vi "MT_Abs.vi"(0 "X轴位置(mm)":dbl, 1 "Y轴位置(mm)":dbl, 3 "Error In":errorcluster caption="错误输入") -> (10 "Error Out":errorcluster caption="错误输出")   [LabVIEW 2020]
uses:
  lib/MT/MT_API.lvlib
panel:
  # "将设备移动到指定位置\n并等待其移动完成"
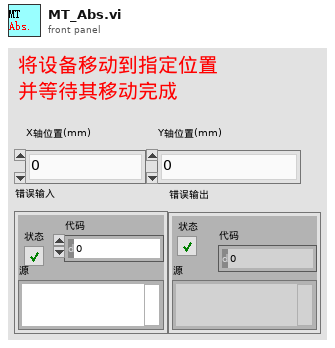
[diagram p1: front panel]
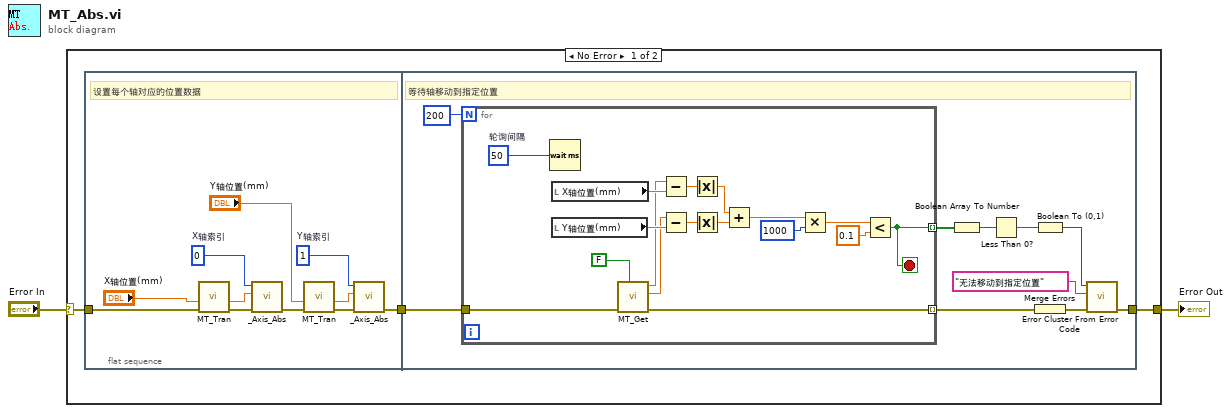
[diagram p0: block diagram]
diagram:
  n1 = case shown="No Error" "Error In" {
    selector: "Error In" -> [w5 w44]
    tunnel: [w3 w44] -> w1
    frame No Error {
      n2 = flat-sequence {
        tunnel: w5 -> [w9]
        tunnel: [w10] -> w4
        tunnel: w4 -> [w26]
        tunnel: [w21] -> w3
        frame #0 {
          w7 = 1  # Y轴索引
          w8 = 0  # X轴索引
          # "设置每个轴对应的位置数据"
          n3 = call "MT_Tran.vi"("Error In"=w9, "位置(mm)"="X轴位置(mm)") -> ("Error Out"=w12:errorcluster, "脉冲位置"=w15:dbl)  [unwired: 6 in, 2 out]
          n4 = call "_Axis_Abs.vi"("Error In"=w12, "绝对位置"=w15, "轴序号"=w8) -> ("Error Out"=w6:errorcluster)  [unwired: 8 in]
          n5 = call "MT_Tran.vi"("Error In"=w6, "位置(mm)"="Y轴位置(mm)") -> ("Error Out"=w11:errorcluster, "脉冲位置"=w13:dbl)  [unwired: 6 in, 2 out]
          n6 = call "_Axis_Abs.vi"("Error In"=w11, "绝对位置"=w13, "轴序号"=w7) -> ("Error Out"=w10:errorcluster)  [unwired: 8 in]
        }
        frame #1 {
          # "等待轴移动到指定位置"
          n7 = for {
            N: 200 -> [_]
            tunnel: w26 -> [w43]
            tunnel: [w35] -> w25 mode=indexing
            tunnel: [w34] -> w23 mode=indexing
            stop <- w35 stop-if-true
            w33 = 50  # 轮询间隔
            n8 = Wait (ms)(milliseconds to wait=w33) -> ()  [unwired: 1 out]
            n9 = local read "X轴位置(mm)"() -> (w42:dbl)
            n10 = local read "Y轴位置(mm)"() -> (w37:dbl)
            n11 = call "MT_Get.vi"("手动操作(False)"=FALSE, "Error In"=w43) -> ("Error Out"=w34:errorcluster, "Y轴位置"=w27:dbl, "X轴位置"=w28:dbl)  [unwired: 5 in, 2 out]
            n12 = Subtract(x=w28, y=w42) -> (x-y=w40:dbl)
            n13 = Subtract(x=w27, y=w37) -> (x-y=w39:dbl)
            n14 = Absolute Value(x=w40) -> (abs(x)=w41:dbl)
            n15 = Absolute Value(x=w39) -> (abs(x)=w38:dbl)
            n16 = Add(x=w41, y=w38) -> (x+y=w31:dbl)
            n17 = Multiply(x=w31, y=1000) -> (x*y=w29:dbl)
            n18 = Less?(x=w29, y=0.1) -> (x < y?=w35:bool)
          }
          n19 = Boolean Array To Number(Boolean array=w25) -> (number=w20:u32)
          n20 = Less Than 0?(x=w20) -> (x < 0?=w19:bool)
          n21 = Boolean To (0,1)(Boolean=w19) -> (0, 1=w18:i16)
          n22 = Merge Errors(w23) -> (w22:errorcluster)
          n23 = call <vilib>:"Error Cluster From Error Code.vi"("error in (no error)"=w22, "error message (\"\")"="无法移动到指定位置", "error code (0)"=w18) -> ("error out"=w21:errorcluster)  [unwired: 6 in]
        }
      }
    }
    frame Error {
    }
  }
  "Error Out" <- w1
